vi "Create Serial Channel Resources.vi"() -> (4 "serial channel resources":T1)   [LabVIEW 2020, in "GettingStarted_Common_148X_FPGA.lvlib"]
uses:
  GettingStarted_Common_148X_FPGA.lvlib
  Types/Serial Channel Resources.ctl
  Types/Single Serial Channel Resources.ctl
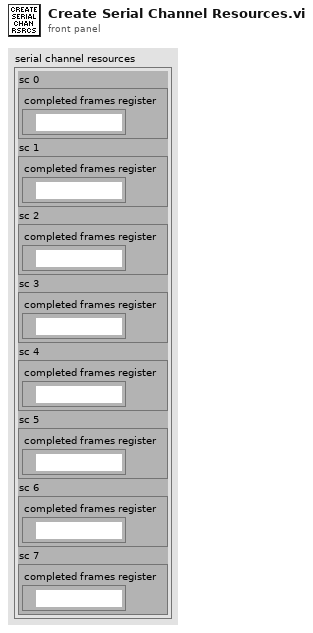
[diagram p1: front panel]
types:
  T1 = typedef "GettingStarted_Common_148X_FPGA.lvlib/Serial Channel Resources.ctl" = cluster{"sc 0":T2, "sc 1":T2, "sc 2":T2, "sc 3":T2, "sc 4":T2, "sc 5":T2, "sc 6":T2, "sc 7":T2}
  T2 = typedef "GettingStarted_Common_148X_FPGA.lvlib/Single Serial Channel Resources.ctl" = cluster{"completed frames register":refnum<k21>}
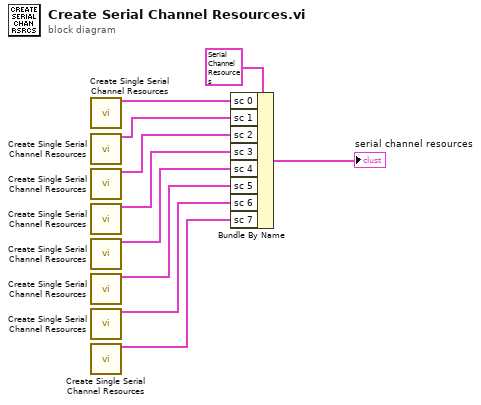
[diagram p0: block diagram]
diagram:
  n1 = call "Create Single Serial Channel Resources.vi"() -> ("single serial channel resources"=w2:T2)  [unwired: 15 in]
  n2 = call "Create Single Serial Channel Resources.vi"() -> ("single serial channel resources"=w3:T2)  [unwired: 15 in]
  n3 = call "Create Single Serial Channel Resources.vi"() -> ("single serial channel resources"=w4:T2)  [unwired: 15 in]
  n4 = call "Create Single Serial Channel Resources.vi"() -> ("single serial channel resources"=w5:T2)  [unwired: 15 in]
  n5 = call "Create Single Serial Channel Resources.vi"() -> ("single serial channel resources"=w7:T2)  [unwired: 15 in]
  n6 = call "Create Single Serial Channel Resources.vi"() -> ("single serial channel resources"=w8:T2)  [unwired: 15 in]
  n7 = call "Create Single Serial Channel Resources.vi"() -> ("single serial channel resources"=w9:T2)  [unwired: 15 in]
  n8 = call "Create Single Serial Channel Resources.vi"() -> ("single serial channel resources"=w10:T2)  [unwired: 15 in]
  n9 = Bundle By Name(cluster=T1 {"sc 0"={"completed frames register"=""}, "sc 1"={"completed frames register"=""}, "sc 2"={"completed frames register"=""}, "sc 3"={"completed frames register"=""}, "sc 4"={"completed frames register"=""}, "sc 5"={"completed frames register"=""}, "sc 6"={"completed frames register"=""}, "sc 7"={"completed frames register"=""}} ("serial channel data resources"), "sc 0"=w2, "sc 1"=w3, "sc 2"=w4, "sc 3"=w5, "sc 4"=w7, "sc 5"=w8, "sc 6"=w9, "sc 7"=w10) -> (→"serial channel resources":T1)
